vi "tlc_Shutdown.vi"(8 "error in (no error)":errorcluster) -> (0 "error out":errorcluster)   [LabVIEW 2018]
uses:
  Controls/tlc_User Interface Data Type.ctl
  Modules/Display/tlc_Display_Command Control.ctl
  Modules/Hardware/tlc_Hardware_Command Control.ctl
  Modules/File/tlc_File_Command Control.ctl
  Modules/Cue/tlc_Cue_Information Command.ctl
panel:
  # "Input"
  # "Output"
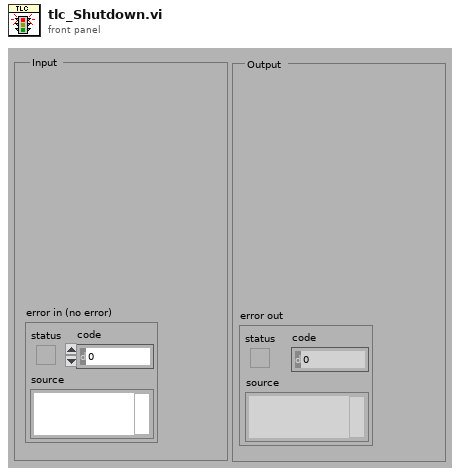
[diagram p1: front panel]
types:
  T1 = typedef "tlc_Cue_Information Command.ctl" = enum16{"Add Cue", "Delete Cue", "Get Cue Values", "Set Cue Values", "Swap", "Get Number of Cues", "Initialize", "Get Empty Cue"}
  T2 = typedef "tlc_File_Command Control.ctl" = enum16{"Initialize", "Save Cues", "Load Cues", "Shutdown"}
  T3 = typedef "tlc_Hardware_Command Control.ctl" = enum16{"Initialize", "Write", "Shutdown"}
  T4 = typedef "tlc_Display_Command Control.ctl" = enum16{"Initialize", "Update UI", "Shutdown"}
  T5 = typedef "tlc_User Interface Data Type.ctl" = enum16{"Initialize", "Initialize Front Panel", "Update Front Panel Channels", "Select Cue in Cue List", "Enable/Disable Front Panel Controls", "Update Cue List", "Stop"}
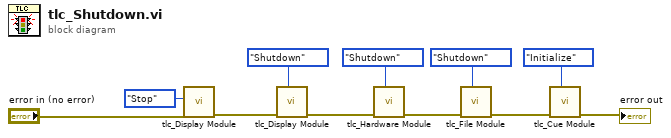
[diagram p0: block diagram]
diagram:
  n1 = call "tlc_Display Module.vi"("error in (no error)"="error in (no error)", "Data Type"=tlc_User_Interface_Data_Type."Stop") -> ("error out"=w9:errorcluster)  [unwired: 9 in]
  n2 = call "tlc_Display Module.vi"("Command (Update UI)"=tlc_Display_Command_Control."Shutdown", "error in (no error)"=w9) -> ("error out"=w6:errorcluster)  [unwired: 9 in]
  n3 = call "tlc_Hardware Module.vi"("Command (Write)"=tlc_Hardware_Command_Control."Shutdown", "error in (no error)"=w6) -> ("error out"=w5:errorcluster)  [unwired: 9 in]
  n4 = call "tlc_File Module.vi"("Command"=tlc_File_Command_Control."Shutdown", "error in (no error)"=w5) -> ("error out"=w4:errorcluster)  [unwired: 8 in, 1 out]
  n5 = call "tlc_Cue Module.vi"("Command"=tlc_Cue_Information_Command."Initialize", "error in (no error)"=w4) -> ("error out"=→"error out":errorcluster)  [unwired: 6 in, 2 out]
